vi "TP 1.3.vi"() -> ()   [LabVIEW 2013]
panel:
  out "Mayor":string
  in  "Nombre":string[](array[string])
  in  "Edad":dbl[](array[numeric])
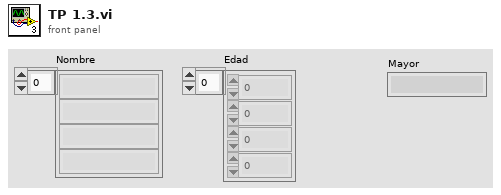
[diagram p1: front panel]
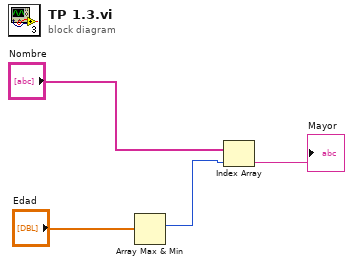
[diagram p0: block diagram]
diagram:
  n1 = Array Max & Min(array="Edad") -> (max index (indices)=w3:i32)  [unwired: 3 out]
  n2 = Index Array(array="Nombre", index=w3) -> (element=→"Mayor":string)
